vi "ScpStop.vi"(8 "error in (no error)":errorcluster, 11 "hDevice in":u32) -> (0 "error out":errorcluster, 2 "Stopped?":bool, 3 "hDevice":u32)   [LabVIEW 2018, in "LibTiePie.lvlib"]
uses:
  LibTiePie.lvlib
  LabViewHS4/libtiepie.dll
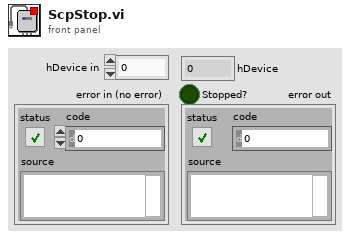
[diagram p1: front panel]
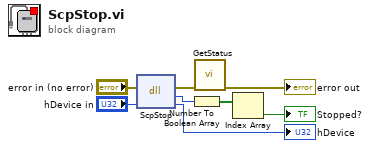
[diagram p0: block diagram]
diagram:
  n1 = dll-call lib="C:/Users/cwaha/Documents/LabViewHS4/libtiepie.dll" fn="ScpStop"(error in="error in (no error)", "hDevice"="hDevice in") -> (error out=w2:errorcluster, "Stopped?"=w5:u8, "hDevice"=→"hDevice":u32)  [unwired: 2 in, 1 out]
  n2 = Number To Boolean Array(number=w5) -> (Boolean array=w4:bool[])
  n3 = call "GetStatus.vi"("error in (no error)"=w2) -> ("error out"=→"error out":errorcluster)  [unwired: 10 in]
  n4 = Index Array(array=w4) -> (element=→"Stopped?":bool)  [unwired: 1 in]
